vi "00 - VISA GPIB TCPIP Serial USB.vi"() -> ()   [LabVIEW 2021]
panel:
  in  "VISA resource name":refnum<visa-resource-name>
  in  "duplicate session (F)":bool
  in  "access mode":u32
  in  "error in (no error)":errorcluster
  in  "VISA Open timeout (0)":u32
  out "error out":errorcluster
  in  "write buffer":string
  out "read buffer":string
  in  "byte count":u32
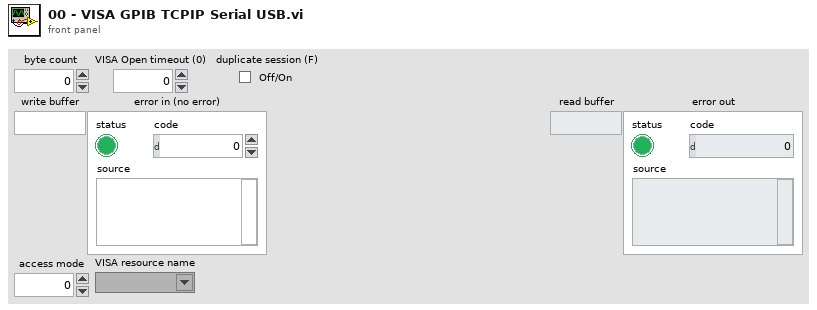
[diagram p1: front panel]
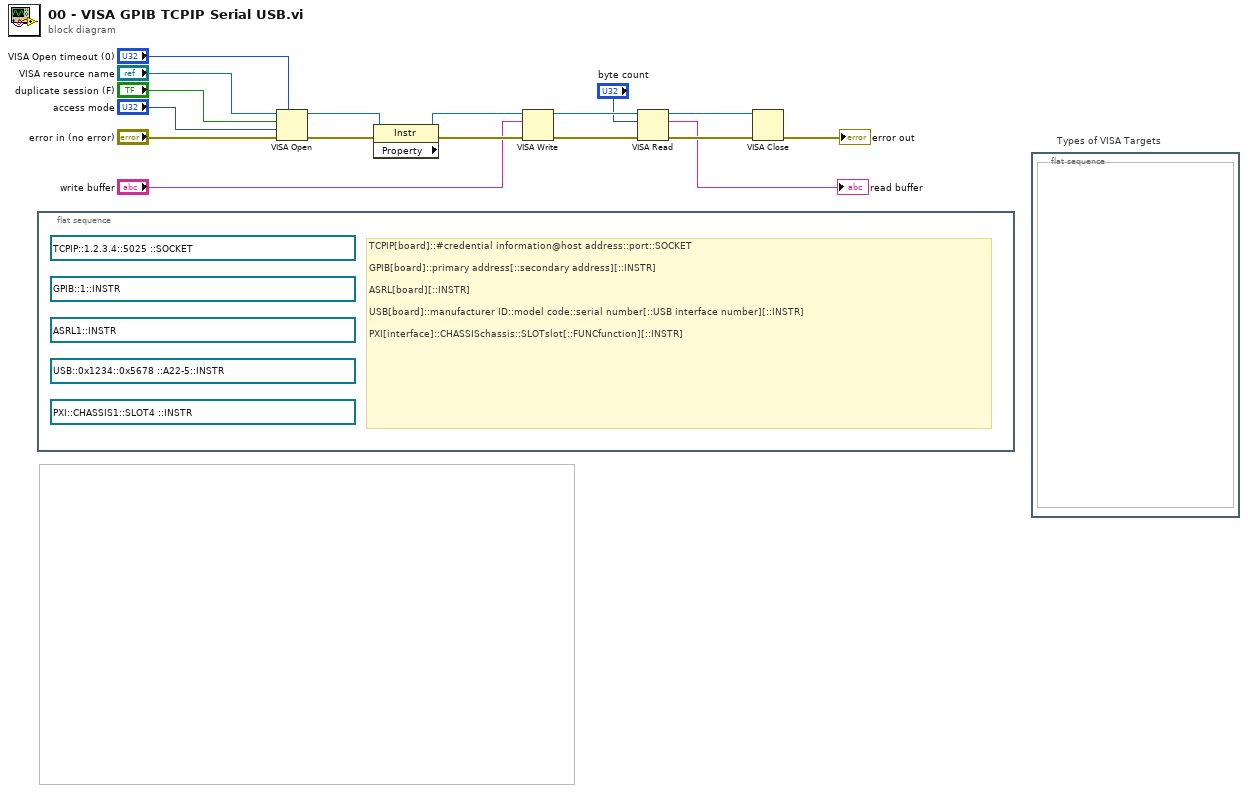
[diagram p0: block diagram]
diagram:
  n1 = flat-sequence {
    frame #0 {
      (unwired) refnum<visa-resource-name> "PXI::CHASSIS1::SLOT4 ::INSTR " ("VISA resource name")
      (unwired) refnum<visa-resource-name> "USB::0x1234::0x5678 ::A22-5::INSTR" ("VISA resource name")
      (unwired) refnum<visa-resource-name> "TCPIP::1.2.3.4::5025 ::SOCKET " ("VISA resource name")
      (unwired) refnum<visa-resource-name> "ASRL1::INSTR " ("VISA resource name")
      (unwired) refnum<visa-resource-name> "GPIB::1::INSTR" ("VISA resource name")
      # "TCPIP[board]::#credential information@host address::port::SOCKET \n\nGPIB[board]::primary address[::secondary address][::INSTR] \n\nASRL[board][::INSTR] \n\nUSB[board]::manufacturer ID::model code::serial number[::USB interface number][::INSTR] \n\nPXI[interface]::CHASSISchassis::SLOTslot[::FUNCfunction][::INSTR]"
    }
  }
  n2 = VISA Open(timeout (0)="VISA Open timeout (0)", duplicate session (F)="duplicate session (F)", access mode="access mode", error in (no error)="error in (no error)", VISA resource name="VISA resource name") -> (VISA resource name=w4:refnum<visa-resource-name>, error out=w13:errorcluster)
  n3 = property class="Instr" props=[](reference=w4, error in=w13) -> (reference out=w3:refnum<visa-resource-name>, error out=w12:errorcluster)  [unwired: 1 out]
  n4 = VISA Write(VISA resource name=w3, write buffer="write buffer", error in (no error)=w12) -> (VISA resource name out=w17:refnum<visa-resource-name>, error out=w16:errorcluster)  [unwired: 1 out]
  n5 = VISA Read(VISA resource name=w17, byte count="byte count", error in (no error)=w16) -> (VISA resource name out=w15:refnum<visa-resource-name>, read buffer=→"read buffer":string, error out=w14:errorcluster)  [unwired: 1 out]
  n6 = VISA Close(VISA resource name=w15, error in (no error)=w14) -> (error out=→"error out":errorcluster)
  n7 = flat-sequence "Types of VISA Targets" {
    frame #0 {
    }
  }
